vi "Day 8-Build Set.vi"(11 "String in":string) -> (3 "Set out":set{string}(c389))   [LabVIEW 2021]
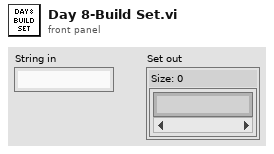
[diagram p1: front panel]
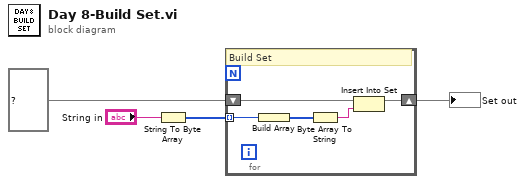
[diagram p0: block diagram]
diagram:
  n1 = String To Byte Array(string="String in") -> (unsigned byte array=w2:u8[])
  n2 = for {
    tunnel: w2 -> [w9] mode=indexing
    shift-right: [w6] -> w4
    shift-left: set{string} {} ("Set in") -> [w5]
    # "Build Set"
    n3 = Build Array(w9) -> (w7:u8[])
    n4 = Byte Array To String(unsigned byte array=w7) -> (string=w8:string)
    n5 = Insert Into Set(10:w8, 11:w5) -> (3:w6:set{string})  [unwired: 1 out]
  }
  "Set out" <- w4
